vi "TDMSAdv deleteCurrFile .vi"(8 "error in (no error)":errorcluster, 11 "TDMSAdv in":refnum<class "TDMSAdv.lvclass">) -> (0 "error out":errorcluster, 3 "TDMSAdv out":refnum<class "TDMSAdv.lvclass">)   [LabVIEW 2018, in "TDMSAdv.lvclass"]
uses:
  TDMSAdv.lvclass
  TDMSAdv.lvclass/TDMSAdv.ctl
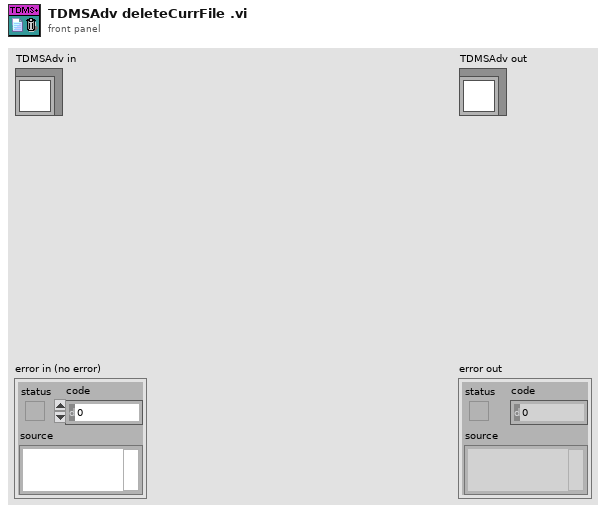
[diagram p1: front panel]
types:
  T1 = enum16{"open", "open or create", "create or replace", "create", "open (read-only)"}
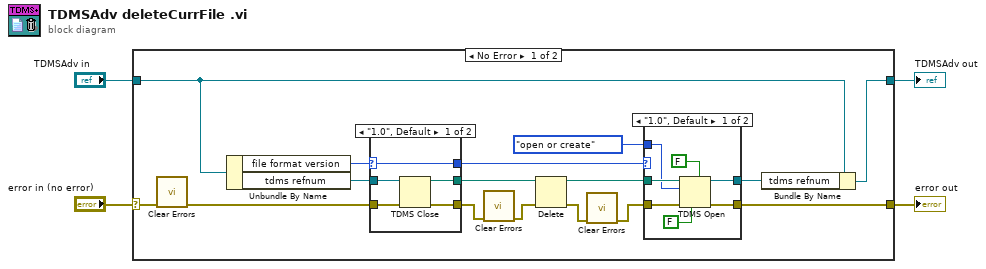
[diagram p0: block diagram]
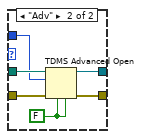
[diagram p2: hidden frame]
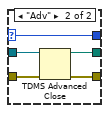
[diagram p3: hidden frame]
diagram:
  n1 = case shown="No Error" "error in (no error)" {
    selector: "error in (no error)" -> [w17 w45]
    tunnel: [w6 w45] -> w3
    tunnel: [w7 w44] -> w1
    tunnel: "TDMSAdv in" -> [w9 w44]
    frame No Error {
      n2 = call <vilib>:"Clear Errors.vi"("error in (no error)"=w17) -> ("error out"=w20:errorcluster)  [unwired: 5 in, 1 out]
      n3 = Unbundle By Name(w9) -> ("file format version"=w18:enum16{"1.0", "2.0", "Adv"}, "tdms refnum"=w19:refnum<k34>)
      n4 = case shown="\"1.0\", Default" w18 {
        selector: w18 -> [w34 w39]
        tunnel: w20 -> [w35 w43]
        tunnel: [w36 w42] -> w15
        tunnel: [w37 w41] -> w16
        tunnel: w19 -> [w38 w40]
        tunnel: [w34 w39] -> w12
        frame "1.0", Default {
          n5 = TDMS Close(8:w35, 11:w38) -> (0:w36:errorcluster, 3:w37:path)
        }
        frame "Adv" {
          n6 = TDMS Advanced Close(8:w43, 11:w40) -> (0:w42:errorcluster, 3:w41:path)  [unwired: 2 in]
        }
      }
      n7 = call <vilib>:"Clear Errors.vi"("error in (no error)"=w15) -> ("error out"=w14:errorcluster)  [unwired: 5 in, 1 out]
      n8 = Delete(path (use dialog)=w16, error in=w14) -> (deleted path=w11:path, error out=w13:errorcluster)  [unwired: 3 in, 1 out]
      n9 = call <vilib>:"Clear Errors.vi"("error in (no error)"=w13) -> ("error out"=w10:errorcluster)  [unwired: 5 in, 1 out]
      n10 = case shown="\"1.0\", Default" w12 {
        tunnel: w10 -> [w24 w33]
        tunnel: [w25 w32] -> w6
        tunnel: [w26 w31] -> w8
        tunnel: w11 -> [w27 w30]
        tunnel: T1."open or create" ("operation (0:open)") -> [w23 w29]
        frame "1.0", Default {
          n11 = TDMS Open(5:FALSE ("create index file? (T)"), 6:FALSE ("disable buffering? (T)"), 8:w24, 10:w23, 11:w27) -> (0:w25:errorcluster, 3:w26:refnum<k34>)  [unwired: 2 in]
        }
        frame "Adv" {
          w28 = FALSE ("enable asynchronous? (T)")
          n12 = TDMS Advanced Open(4:w28, 6:w28, 8:w33, 10:w29, 11:w30) -> (0:w32:errorcluster, 3:w31:refnum<k34>)  [unwired: 1 out]
        }
      }
      n13 = Bundle By Name(cluster=w9, "tdms refnum"=w8) -> (w7:refnum<class "TDMSAdv.lvclass">)
    }
    frame Error {
    }
  }
  "error out" <- w3
  "TDMSAdv out" <- w1
